vi "FFT module.vi"(0 "h_signal":u16[][](array[numeric]), 1 "Alines":i32, 5 "h_trimmed_signal in":sgl[](array[numeric]), 7 "curve":u16[](array[numeric]), 9 "Save  parameters":T1={"start pixel"=0, "#pixels to save"=300}, 11 "error in":errorcluster) -> (6 "h_trimmed_signal out":sgl[](array[numeric]), 15 "error out":errorcluster)   [LabVIEW 2018]
uses:
  DLL/CUDA_FFT_2_channel_ref_ret_fast.dll
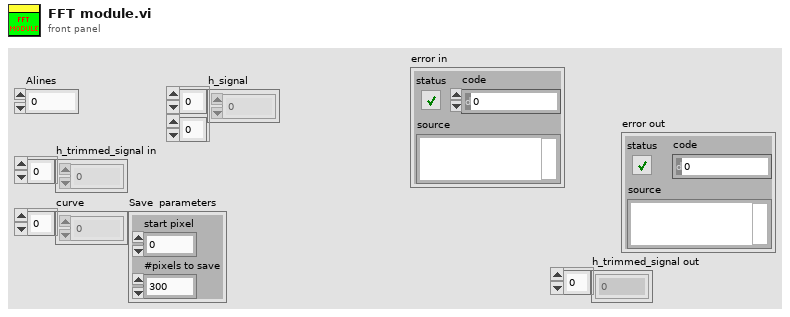
[diagram p1: front panel]
types:
  T1 = cluster{"start pixel":i32, "#pixels to save":i32}
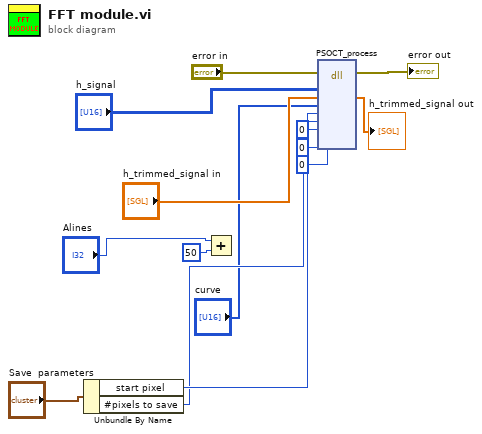
[diagram p0: block diagram]
diagram:
  n1 = Unbundle By Name("Save  parameters") -> ("start pixel"=w7:i32, "#pixels to save"=w6:i32)
  n2 = Add(x="Alines", y=50) -> ()  [unwired: 1 out]
  n3 = dll-call lib="C:/Project/SerialSectionOCT/SerialSectOCT/Labview Software/DLL/CUDA_FFT_2_channel_ref_ret_fast.dll" fn="PSOCT_process"(error in="error in", "h_signal"="h_signal", "h_processed_ref"="h_trimmed_signal in", "h_processed_ret"="curve", "z0"=w7, "depth"=w6, "NALINES"=0, "NBLINES"=0, "SAMPLES"=0) -> (error out=→"error out":errorcluster, "h_processed_ref"=→"h_trimmed_signal out":sgl[])  [unwired: 10 in, 1 out]
